vi "hmi_cheesy_drive.vi"(9 "Quick Turn":bool, 10 "Wheel":dbl, 11 "Throttle":dbl) -> (3 "Drive Data":cluster{"Left":dbl, "Right":dbl})   [LabVIEW 2011]
uses:
  drivetrain/drivetrain_globals.vi
panel:
  in  "Speedturn_Sens_High":dbl=1.7
  in  "Quickturn_Sens_High":dbl=1.0
  in  "Speedturn_Sens_Low":dbl=1.5
  in  "Quickturn_Sens_Low":dbl=1.2
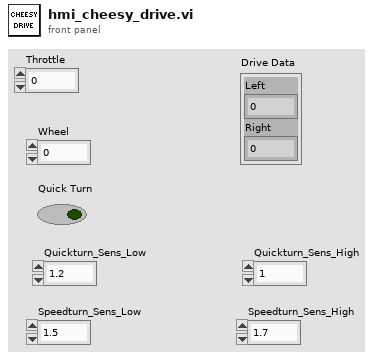
[diagram p1: front panel]
types:
  T1 = typedef "gear_shift_state.ctl" = enum16{"low", "high"}
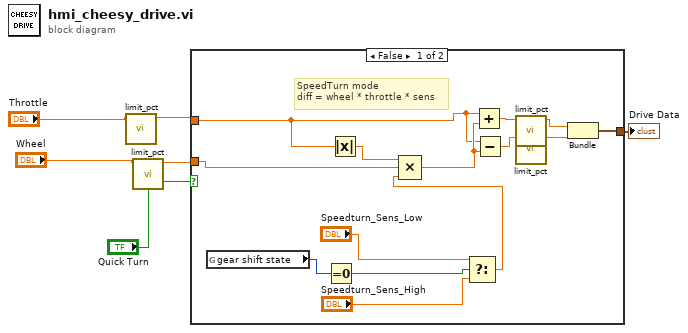
[diagram p0: block diagram]
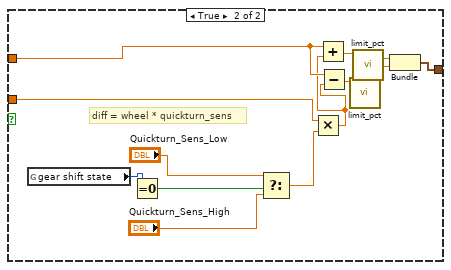
[diagram p2: hidden frame]
diagram:
  n1 = call "limit_pct.vi"("PCT"="Throttle") -> ("PCT Out"=w3:dbl)  [unwired: 10 in]
  n2 = call "limit_pct.vi"("PCT"="Wheel") -> ("PCT Out"=w1:dbl)  [unwired: 10 in]
  n3 = case shown="False" "Quick Turn" {
    tunnel: w1 -> [w17 w29]
    tunnel: w3 -> [w8 w28]
    tunnel: [w14 w26] -> w5
    frame False {
      # "SpeedTurn mode\ndiff = wheel * throttle * sens"
      n4 = global read "drivetrain_globals.vi" "gear shift state"() -> (w7:T1)
      n5 = Equal To 0?(x=w7) -> (x = 0?=w20:bool)
      n6 = Absolute Value(x=w8) -> (abs(x)=w9:dbl)
      n7 = Select(t="Speedturn_Sens_Low", s=w20, f="Speedturn_Sens_High") -> (s? t:f=w16:dbl)
      n8 = Compound Arithmetic op=MULTIPLY(w9, w17, w16) -> (w15:dbl)
      n9 = Add(x=w8, y=w15) -> (x+y=w12:dbl)
      n10 = Subtract(x=w8, y=w15) -> (x-y=w11:dbl)
      n11 = call "limit_pct.vi"("PCT"=w12) -> ("PCT Out"=w13:dbl)  [unwired: 10 in]
      n12 = call "limit_pct.vi"("PCT"=w11) -> ("PCT Out"=w10:dbl)  [unwired: 10 in]
      n13 = Bundle("PCT Out"=w13, "PCT Out"=w10) -> (w14:cluster{"PCT Out":dbl, "PCT Out":dbl})  [unwired: 1 in]
    }
    frame True {
      # "diff = wheel * quickturn_sens"
      n14 = global read "drivetrain_globals.vi" "gear shift state"() -> (w21:T1)
      n15 = Equal To 0?(x=w21) -> (x = 0?=w31:bool)
      n16 = Select(t="Quickturn_Sens_Low", s=w31, f="Quickturn_Sens_High") -> (s? t:f=w30:dbl)
      n17 = Multiply(x=w29, y=w30) -> (x*y=w27:dbl)
      n18 = Add(x=w28, y=w27) -> (x+y=w24:dbl)
      n19 = Subtract(x=w28, y=w27) -> (x-y=w22:dbl)
      n20 = call "limit_pct.vi"("PCT"=w22) -> ("PCT Out"=w23:dbl)  [unwired: 10 in]
      n21 = call "limit_pct.vi"("PCT"=w24) -> ("PCT Out"=w25:dbl)  [unwired: 10 in]
      n22 = Bundle("PCT Out"=w25, "PCT Out"=w23) -> (w26:cluster{"PCT Out":dbl, "PCT Out":dbl})  [unwired: 1 in]
    }
  }
  "Drive Data" <- w5
